vi "get Session Prefix.vi"(7 "Remote Connection Session":refnum<class "Remote Connection Session.lvclass">) -> (8 "Session Prefix":string)   [LabVIEW 2012, in "REx.lvlib" / "Remote Connection Session.lvclass"]
uses:
  Remote Connection Session.lvclass
  <userlib>/_Session Fwk/Session - Root.lvclass
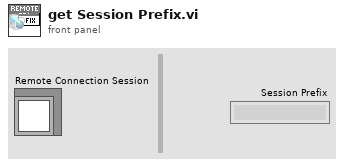
[diagram p1: front panel]
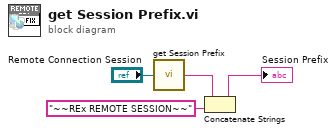
[diagram p0: block diagram]
diagram:
  n1 = call-parent "get Session Prefix.vi"("Session - Root"="Remote Connection Session") -> ("Session Prefix"=w3:string)  [unwired: 14 in]
  n2 = Concatenate Strings(w3, "~~REx REMOTE SESSION~~" ("string")) -> (→"Session Prefix":string)
